vi "ValueSignalByPathArray.vi"(0 "VI Reference In":refnum<vi>, 5 "Control Path":string[](array[string]), 7 "Value (Signaling)":variant, 11 "error in":errorcluster) -> (4 "VI Reference Out":refnum<vi>, 15 "error out":errorcluster)   [LabVIEW 2016, in "Drona.lvlib" / "ValueSignal.lvlib"]
doc: "<b>Sets the value of controlsI.</b>\n\nThe path of the control should be given in the successive index of the array"
uses:
  ValueSignal.lvlib
  Setup/GetControlRef/GetControlRef.lvlib
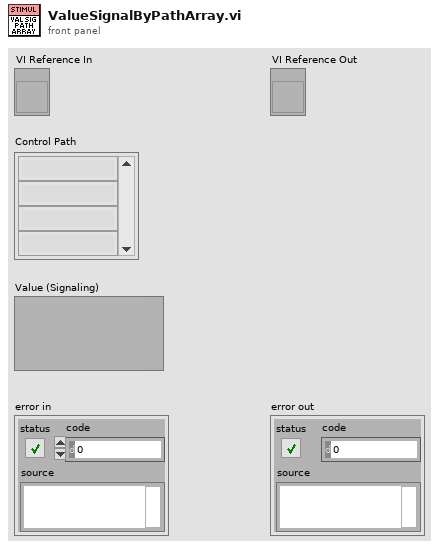
[diagram p1: front panel]
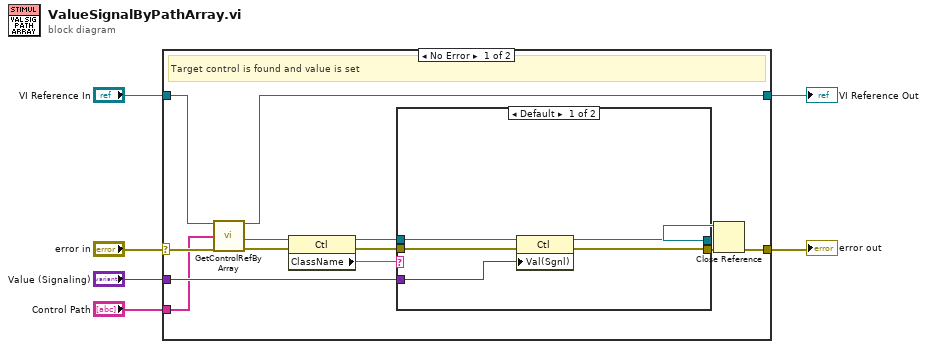
[diagram p0: block diagram]
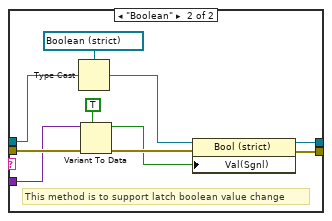
[diagram p2: hidden frame]
diagram:
  n1 = case shown="No Error" "error in" {
    selector: "error in" -> [w18 w36]
    tunnel: "Control Path" -> [w15 _]
    tunnel: "VI Reference In" -> [w14 w35]
    tunnel: [w13 w35] -> w3
    tunnel: "Value (Signaling)" -> [w19 _]
    tunnel: [w12 w36] -> w1
    frame No Error {
      # "Target control is found and value is set"
      n2 = call "GetControlRefByArray.vi"("VI Reference In"=w14, "Control Path"=w15, "error In"=w18) -> ("VI Reference Out"=w13:refnum<vi>, "Ctl Refnum"=w9:refnum<vi>, "error out"=w17:errorcluster)  [unwired: 10 in]
      n3 = property class="Ctl"(reference=w9, error in=w17) -> (reference out=w7:refnum<vi>, error out=w10:errorcluster, "ClassName"=w8:string)
      n4 = case shown="Default" w8 {
        tunnel: w19 -> [w21 w26]
        tunnel: w10 -> [w24 w29]
        tunnel: [w23 w34] -> w16
        tunnel: [w20 w33] -> w11
        tunnel: w7 -> [w22 w31]
        frame Default {
          n5 = property class="Ctl"(reference=w22, error in=w24, "Val(Sgnl)"=w21) -> (reference out=w20:refnum<vi>, error out=w23:errorcluster)
        }
        frame "Boolean" {
          # "This method is to support latch boolean value change"
          n6 = Type Cast(type=refnum<vi> refnum ("OK"), x=w31) -> (*(type *) &x=w30:refnum<vi>)
          n7 = Variant To Data(error in=w29, type=TRUE, Variant=w26) -> (data=w25:bool, error out=w28:errorcluster)
          n8 = property class="Bool (strict)"(reference=w30, error in=w28, "Val(Sgnl)"=w25) -> (reference out=w33:refnum<vi>, error out=w34:errorcluster)
        }
      }
      n9 = Close Reference(reference=w11, error in (no error)=w16) -> (error out=w12:errorcluster)
    }
    frame Error {
    }
  }
  "error out" <- w1
  "VI Reference Out" <- w3
